vi "Connect.vi"(8 "error in (no error)":errorcluster, 11 "reference in":refnum<class "NS master.lvclass">) -> (0 "error out":errorcluster, 3 "reference out":refnum<class "NS master.lvclass">)   [LabVIEW 2019, in "CommandResponse communication.lvlib" / "NS master.lvclass"]
doc: "Connects to Slave device and established network streams communication"
uses:
  NS master.lvclass
  C:/Barkhausen mmWave radar/Development/LV/Barkhausen mmWave hardware control/Host/Intertarget communication/CR_master_class/CR_master.lvclass
  ITC command.ctl
  ITC response.ctl
  CommandResponse communication.lvlib
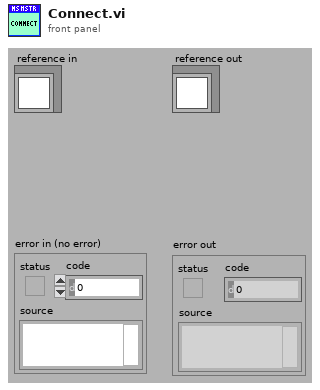
[diagram p1: front panel]
types:
  T1 = typedef "CommandResponse communication.lvlib/ITC response.ctl" = cluster{"status":string, "reponse":string, "data":variant}
  T2 = typedef "CommandResponse communication.lvlib/ITC command.ctl" = cluster{"message":string, "parameters":string, "data":variant}
  T3 = typedef "CommandResponse communication.lvlib/NS master.lvclass/ObjectAttributesRef.ctl" = refnum<data-value>
  T4 = typedef "CommandResponse communication.lvlib/NS master.lvclass/ObjectAttributes.ctl" = cluster{"connected":bool, "stop":bool, "ID":string, "command wr":refnum<k21>, "response rd":refnum<k21>, "data rd":refnum<k21>, "slave ip":string, "slave id":string}
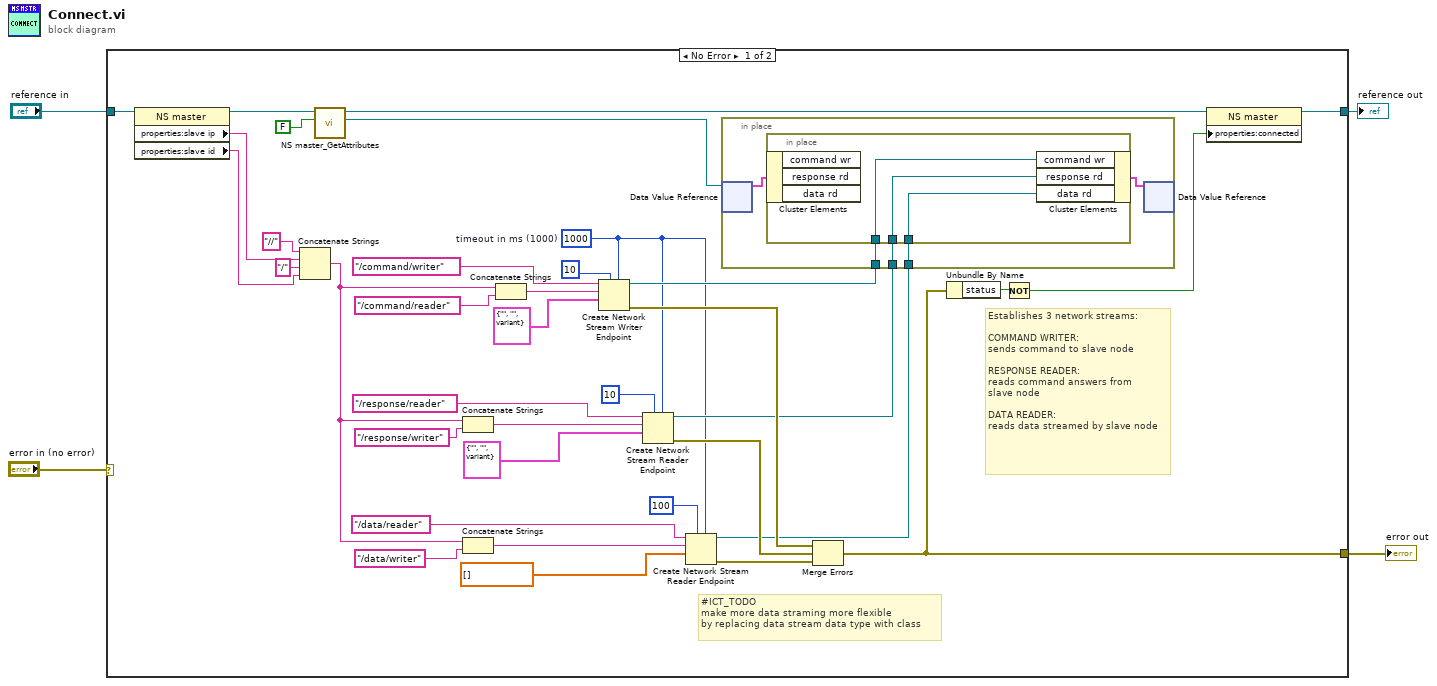
[diagram p0: block diagram]
diagram:
  n1 = case shown="No Error" "error in (no error)" {
    selector: "error in (no error)" -> [_ w50]
    tunnel: [w7 w50] -> w3
    tunnel: [w6 w49] -> w1
    tunnel: "reference in" -> [w39 w49]
    frame No Error {
      w13 = 1000  # timeout in ms (1000)
      # "#ICT_TODO\nmake more data straming more flexible\nby replacing data stream data type with class"
      # "Establishes 3 network streams:\n\nCOMMAND WRITER:\nsends command to slave node\n\nRESPONSE READER:\nreads command answers from\nslave node\n\nDATA READER:\nreads data streamed by slave node"
      n2 = property class="NS master"(reference=w39) -> (reference out=w11:refnum<class "NS master.lvclass">, "properties:slave ip"=w10:string, "properties:slave id"=w9:string)  [unwired: 1 in, 1 out]
      n3 = Concatenate Strings("//" ("reader url"), w10, "/" ("string"), w9) -> (w22:string)
      n4 = call "NS master_GetAttributes.vi"("return data? (T)"=FALSE, "reference in"=w11) -> ("attributes ref"=w17:T3, "reference out"=w40:refnum<class "NS master.lvclass">)  [unwired: 6 in, 2 out]
      n5 = Concatenate Strings(w22, "/response/writer" ("reader url")) -> (w29:string)
      n6 = Concatenate Strings(w22, "/data/writer" ("reader url")) -> (w25:string)
      n7 = Concatenate Strings(w22, "/command/reader" ("reader url")) -> (w37:string)
      n8 = Create Network Stream Writer Endpoint(5:w13, 7:10 ("writer buffer size"), 9:T2 {"message"="", "parameters"="", "data"=variant} ("command"), 10:w37, 11:"/command/writer" ("writer name")) -> (0:w18:errorcluster, 3:w16:refnum<k21>)  [unwired: 2 in]
      n9 = Create Network Stream Reader Endpoint(5:w13, 7:10 ("reader buffer size"), 9:T1 {"status"="", "reponse"="", "data"=variant(cluster{"Boolean Round":bool, "code":i32, "source":string} {"Boolean Round"=FALSE, "code"=0, "source"=""})} ("ITC response"), 10:w29, 11:"/response/reader" ("writer name")) -> (0:w19:errorcluster, 3:w15:refnum<k21>)  [unwired: 2 in]
      n10 = Create Network Stream Reader Endpoint(5:w13, 7:100 ("reader buffer size"), 9:cdb[] [] ("data"), 10:w25, 11:"/data/reader" ("writer name")) -> (0:w20:errorcluster, 3:w14:refnum<k21>)  [unwired: 2 in]
      n11 = in-place {
        in-place-border: w16 -> [w43]
        in-place-border: w15 -> [w42]
        in-place-border: w14 -> [w41]
        n12 = in-place-dvr #1(w17) -> (w45:T4)  [unwired: 1 out]
        n13 = in-place {
          in-place-border: w43 -> [w48]
          in-place-border: w42 -> [w47]
          in-place-border: w41 -> [w46]
          n14 = in-place-cluster #2(w45) -> ()  [unwired: 3 out]
          n15 = in-place-cluster #2("command wr"=w48, "response rd"=w47, "data rd"=w46) -> (w44:T4)
        }
        n16 = in-place-dvr #1(w44) -> ()  [unwired: 2 out]
      }
      n17 = Merge Errors(w18, w19, w20) -> (w7:errorcluster)
      n18 = Unbundle By Name(w7) -> ("status"=w8:bool)
      n19 = Not(x=w8) -> (.not. x?=w5:bool)
      n20 = property class="NS master"(reference=w40, "properties:connected"=w5) -> (reference out=w6:refnum<class "NS master.lvclass">)  [unwired: 1 in, 1 out]
    }
    frame Error {
    }
  }
  "error out" <- w3
  "reference out" <- w1
